vi "VG_ARDUINO.vi"() -> ()   [LabVIEW 2020]
panel:
  in  "ARDUINO":string
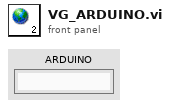
[diagram p1: front panel]
diagram:
